vi "Result_Test.vi"(8 "error in (no error)":errorcluster caption="entrée d'erreur (pas d'erreur)", 11 "Delay en entrée":refnum<class "Operator_Information.lvclass">) -> (0 "error out":errorcluster caption="sortie d'erreur", 3 "Delay en sortie":refnum<class "Operator_Information.lvclass">)   [LabVIEW 2020, in "Library Test.lvlib" / "Operator_Information.lvclass"]
uses:
  Operator_Information.lvclass
  C:/Users/ngarcin/OneDrive - Altyor/Standard TB/Class/Test/Test (Default)/Test (Default).lvclass
  Test_Without_Instr/Test_Without_Inst.lvclass
  Operator_Information.lvclass/Operator_Information.ctl
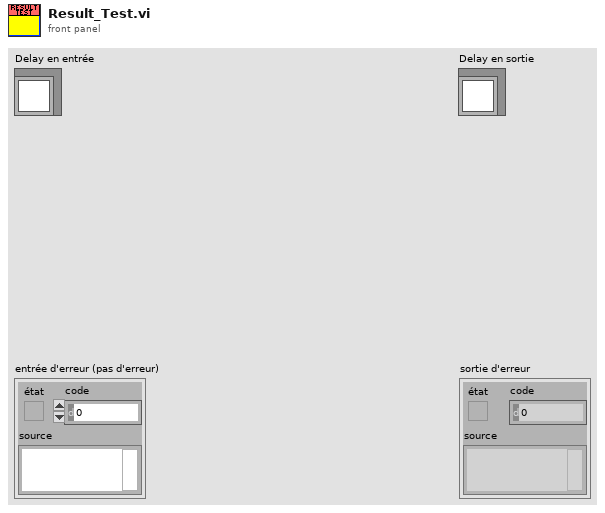
[diagram p1: front panel]
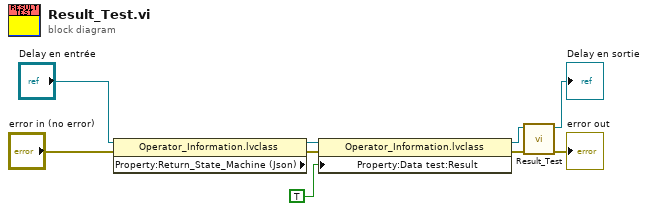
[diagram p0: block diagram]
diagram:
  n1 = property class="Operator_Information.lvclass" props=["Property:Return_State_Machine (Json)"](reference="Delay en entrée", error in="error in (no error)") -> (reference out=w3:refnum<class "Operator_Information.lvclass">, error out=w5:errorcluster)  [unwired: 1 out]
  n2 = property class="Operator_Information.lvclass"(reference=w3, error in=w5, "Property:Data test:Result"=TRUE ("Result")) -> (reference out=w2:refnum<class "Operator_Information.lvclass">, error out=w4:errorcluster)
  n3 = call-parent "Result_Test.vi"("error in (no error)"=w4, "Test_Without_Inst en entrée"=w2) -> ("error out"=→"error out":errorcluster, "Test_Without_Inst en sortie"=→"Delay en sortie":refnum<class "Operator_Information.lvclass">)  [unwired: 8 in]
